vi "average safe distance.vi"(6 "Back Right":dbl, 7 "Front Right":dbl, 8 "Back Left":dbl, 9 "Front Left":dbl) -> (0 "Right Distance":dbl, 1 "Average Absolute Distance":dbl, 2 "Average Distance":dbl, 3 "Left Distance":dbl)   [LabVIEW 2014]
panel:
  # "Distance Inputs"
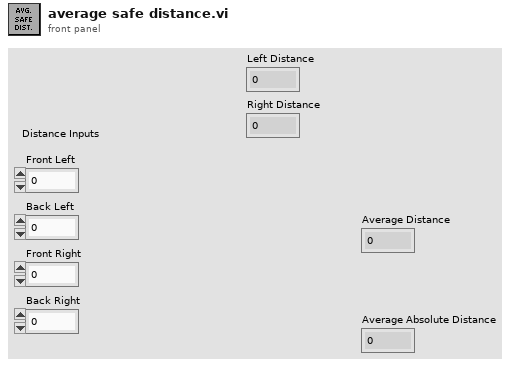
[diagram p1: front panel]
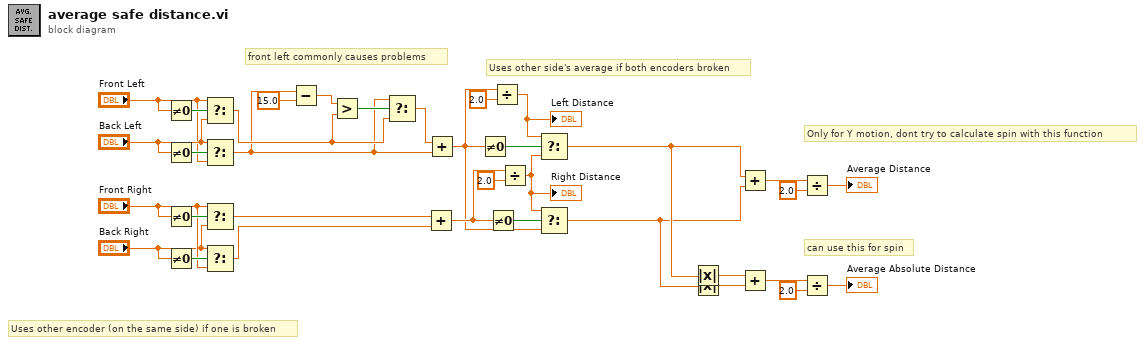
[diagram p0: block diagram]
diagram:
  # "front left commonly causes problems"
  # "can use this for spin"
  # "Only for Y motion, dont try to calculate spin with this function"
  # "Uses other encoder (on the same side) if one is broken"
  # "Uses other side's average if both encoders broken"
  n1 = Not Equal To 0?(x="Front Left") -> (x != 0?=w31:bool)
  n2 = Not Equal To 0?(x="Back Left") -> (x != 0?=w32:bool)
  n3 = Not Equal To 0?(x="Front Right") -> (x != 0?=w33:bool)
  n4 = Not Equal To 0?(x="Back Right") -> (x != 0?=w34:bool)
  n5 = Select(t="Front Left", s=w31, f="Back Left") -> (s? t:f=w3:dbl)
  n6 = Select(t="Back Left", s=w32, f="Front Left") -> (s? t:f=w2:dbl)
  n7 = Select(t="Front Right", s=w33, f="Back Right") -> (s? t:f=w23:dbl)
  n8 = Select(t="Back Right", s=w34, f="Front Right") -> (s? t:f=w22:dbl)
  n9 = Subtract(x=w2, y=15.0) -> (x-y=w5:dbl)
  n10 = Greater?(x=w5, y=w3) -> (0:w4:bool)
  n11 = Select(t=w2, s=w4, f=w3) -> (s? t:f=w1:dbl)
  n12 = Add(x=w23, y=w22) -> (x+y=w19:dbl)
  n13 = Add(x=w1, y=w2) -> (x+y=w17:dbl)
  n14 = Not Equal To 0?(x=w17) -> (x != 0?=w26:bool)
  n15 = Not Equal To 0?(x=w19) -> (x != 0?=w20:bool)
  n16 = Divide(x=w17, y=2.0) -> (x/y=w24:dbl)
  "Left Distance" <- w24
  n17 = Divide(x=w19, y=2.0) -> (x/y=w18:dbl)
  "Right Distance" <- w18
  n18 = Select(t=w24, s=w26, f=w18) -> (s? t:f=w10:dbl)
  n19 = Select(t=w18, s=w20, f=w17) -> (s? t:f=w9:dbl)
  n20 = Absolute Value(x=w10) -> (abs(x)=w8:dbl)
  n21 = Absolute Value(x=w9) -> (abs(x)=w7:dbl)
  n22 = Add(x=w10, y=w9) -> (x+y=w16:dbl)
  n23 = Add(x=w8, y=w7) -> (x+y=w11:dbl)
  n24 = Divide(x=w16, y=2.0) -> (x/y=→"Average Distance":dbl)
  n25 = Divide(x=w11, y=2.0) -> (x/y=→"Average Absolute Distance":dbl)
